vi "Save FP Object Configuration.vi"(8 "error in (no error)":errorcluster, 9 "High Level Config Settings":T1, 10 "Objects Configurations":T2[](array[typedef]), 11 "VI Identifier":string) -> (0 "error out":errorcluster)   [LabVIEW 2017, in "Front Panel Publisher.lvlib" / "Web Front Panel.lvclass"]
uses:
  Web Front Panel.lvclass
  Controls/FP Object Configuration.ctl
  Controls/All Config Settings.ctl
  Controls/High Level Config Settings.ctl
  Front Panel Manager_class/Front Panel Manager.lvclass
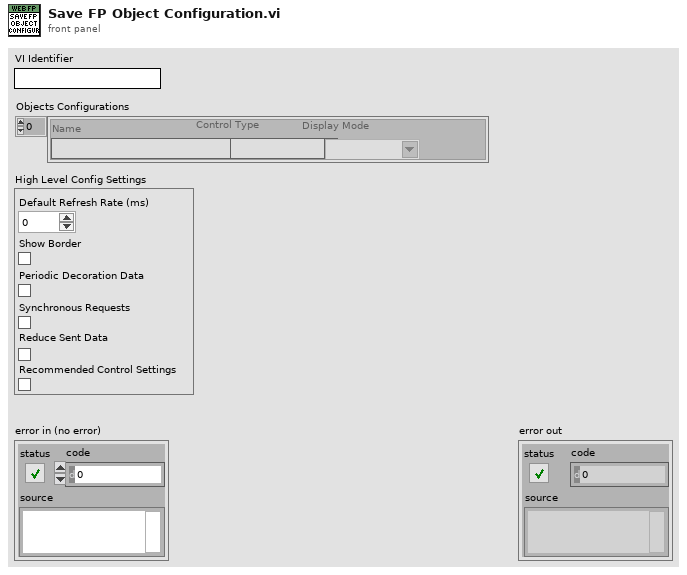
[diagram p1: front panel]
types:
  T1 = typedef "Front Panel Publisher.lvlib/Web Front Panel.lvclass/High Level Config Settings.ctl" = cluster{"Default Refresh Rate (ms)":i32, "Show Border":bool, "Periodic Decoration Data":bool, "Synchronous Requests":bool, "Reduce Sent Data":bool, "Recommended Control Settings":bool}
  T2 = typedef "Front Panel Publisher.lvlib/Web Front Panel.lvclass/FP Object Configuration.ctl" = cluster{"Name":string, "Control Type":string, "Display Mode":string}
  T3 = typedef "Front Panel Publisher.lvlib/Web Front Panel.lvclass/All Config Settings.ctl" = cluster{"Objects Configurations":T2[], "High Level Config Settings":T1}
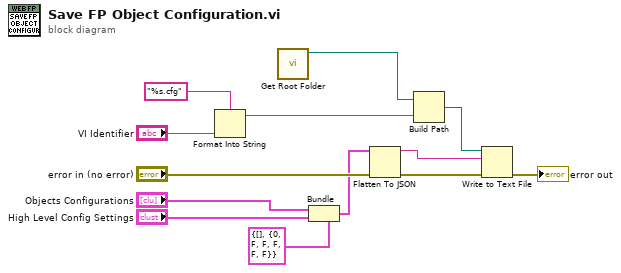
[diagram p0: block diagram]
diagram:
  n1 = Format Into String(format string="%s.cfg", "VI Identifier") -> (resulting string=w2:string)  [unwired: 2 in, 1 out]
  n2 = call "Get Root Folder.vi"() -> ("Root folder"=w1:path)  [unwired: 11 in]
  n3 = Bundle(cluster=T3 {"Objects Configurations"=[], "High Level Config Settings"={"Default Refresh Rate (ms)"=0, "Show Border"=FALSE, "Periodic Decoration Data"=FALSE, "Synchronous Requests"=FALSE, "Reduce Sent Data"=FALSE, "Recommended Control Settings"=FALSE}} ("output cluster"), "Objects Configurations"="Objects Configurations", "High Level Config Settings"="High Level Config Settings") -> (w6:T3)
  n4 = Flatten To JSON(anything=w6, error in (no error)="error in (no error)") -> (JSON string=w9:string, 11:w10:errorcluster)  [unwired: 1 in]
  n5 = Build Path(base path=w1, name or relative path=w2) -> (appended path=w3:path)
  n6 = Write to Text File(file (use dialog)=w3, text=w9, error in=w10) -> (error out=→"error out":errorcluster)  [unwired: 1 in, 2 out]
